vi "SRV_Queue Streaming Halt and Restore States.vi"(8 "error in (no error)":errorcluster, 10 "Commands":T1[](array[typedef]), 11 "Control Queue":refnum<queue>) -> (0 "error out":errorcluster, 3 "Control Queue out":refnum<queue>)   [LabVIEW 2014]
uses:
  Support/SRV_Command-Data Queue Data Type.ctl
  SRV_Streaming Modes.ctl
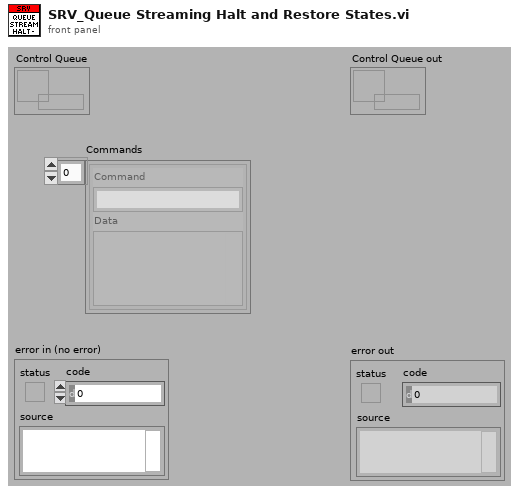
[diagram p1: front panel]
types:
  T1 = typedef "SRV_Command-Data Queue Data Type.ctl" = cluster{"Command":string, "Data":variant}
  T2 = typedef "SRV_Streaming Modes.ctl" = enum16{"Video", "Sensors"}
  T3 = typedef "SRV_Streaming States.ctl" = cluster{"Video":T4, "Sensors":T4}
  T4 = typedef "SRV_Streaming State.ctl" = cluster{"Enabled":bool, "Data":string}
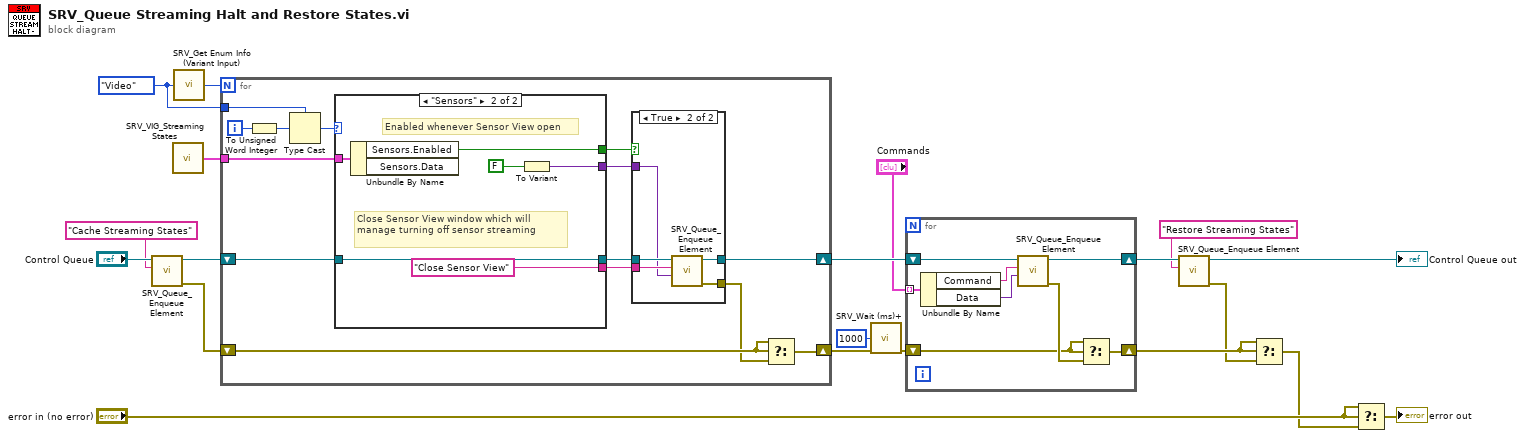
[diagram p0: block diagram]
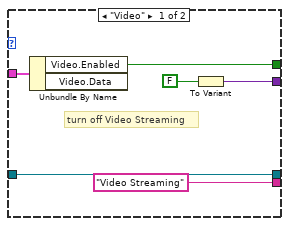
[diagram p2: hidden frame]
diagram:
  w14 = SRV_Streaming_Modes."Video" ("Streaming Modes")
  n1 = call "SRV_Queue_Enqueue Element.vi"("Command"="Cache Streaming States" ("name (unnamed)"), "Command-Data Queue"="Control Queue") -> ("error out"=w12:errorcluster, "Command-Data Queue out"=w16:refnum<queue>)  [unwired: 7 in, 1 out]
  n2 = call "SRV_VIG_Streaming States.vi"() -> ("Streaming States out"=w13:T3)  [unwired: 15 in]
  n3 = call "SRV_Get Enum Info (Variant Input).vi"("Variant (Enum)"=w14) -> ("Enum Size"=w15:i32)  [unwired: 4 in, 2 out]
  n4 = for {
    N: w15 -> [_]
    shift-right: [w34] -> w11
    shift-left: w16 -> [w28]
    tunnel: w14 -> [w31]
    tunnel: w13 -> [w29]
    shift-right: [w21] -> w3
    shift-left: w12 -> [w23]
    i -> [w33]
    n5 = To Unsigned Word Integer(number=w33) -> (unsigned 16bit integer=w32:u16)
    n6 = Type Cast(type=w31, x=w32) -> (*(type *) &x=w30:T2)
    n7 = case shown="\"Sensors\"" w30 {
      tunnel: w29 -> [w40 w46]
      tunnel: w28 -> [w39 w45]
      tunnel: [w39 w45] -> w27
      tunnel: [w38 w41] -> w26
      tunnel: ["Video Streaming" ("Command") "Close Sensor View" ("Command")] -> w25
      tunnel: [w36 w43] -> w24
      frame "Video" {
        # "turn off Video Streaming"
        n8 = Unbundle By Name(w40) -> ("Video.Enabled"=w38:bool)  [unwired: 1 out]
        n9 = To Variant(anything=FALSE ("Show Image")) -> (Variant=w36:variant)
      }
      frame "Sensors" {
        # "Enabled whenever Sensor View open"
        # "Close Sensor View window which will manage turning off sensor streaming"
        n10 = Unbundle By Name(w46) -> ("Sensors.Enabled"=w41:bool)  [unwired: 1 out]
        n11 = To Variant(anything=FALSE ("Show Image")) -> (Variant=w43:variant)
      }
    }
    n12 = case shown="True" w26 {
      tunnel: w27 -> [w47 w52]
      tunnel: [w47 w51] -> w34
      tunnel: w25 -> [_ w50]
      tunnel: w24 -> [_ w49]
      tunnel: [_ w48] -> w22
      frame False {
      }
      frame True {
        n13 = call "SRV_Queue_Enqueue Element.vi"("Data"=w49, "Command"=w50, "Command-Data Queue"=w52) -> ("error out"=w48:errorcluster, "Command-Data Queue out"=w51:refnum<queue>)  [unwired: 6 in, 1 out]
      }
    }
    n14 = Select(t=w23, s=w23, f=w22) -> (s? t:f=w21:errorcluster)
  }
  n15 = call "SRV_Wait (ms)+.vi"("milliseconds to wait"=u32 1000, "error in (no error)"=w3) -> ("error out"=w2:errorcluster)  [unwired: 12 in, 1 out]
  n16 = for {
    shift-right: [w59] -> w9
    shift-left: w11 -> [w60]
    shift-right: [w56] -> w7
    shift-left: w2 -> [w57]
    tunnel: "Commands" -> [w55] mode=indexing
    n17 = Unbundle By Name(w55) -> ("Command"=w54:string, "Data"=w53:variant)
    n18 = call "SRV_Queue_Enqueue Element.vi"("Data"=w53, "Command"=w54, "Command-Data Queue"=w60) -> ("error out"=w58:errorcluster, "Command-Data Queue out"=w59:refnum<queue>)  [unwired: 6 in, 1 out]
    n19 = Select(t=w57, s=w57, f=w58) -> (s? t:f=w56:errorcluster)
  }
  n20 = call "SRV_Queue_Enqueue Element.vi"("Command"="Restore Streaming States", "Command-Data Queue"=w9) -> ("error out"=w6:errorcluster, "Command-Data Queue out"=→"Control Queue out":refnum<queue>)  [unwired: 7 in, 1 out]
  n21 = Select(t=w7, s=w7, f=w6) -> (s? t:f=w5:errorcluster)
  n22 = Select(t="error in (no error)", s="error in (no error)", f=w5) -> (s? t:f=→"error out":errorcluster)
